vi "Read s4 channel status.vi"(8 "error in (no error)":errorcluster, 11 "SPARC4_Channel in":refnum<class "SPARC4_Channel.lvclass">) -> (0 "error out":errorcluster, 1 "channel status":T1, 2 "s4 channel status":T2, 3 "SPARC4_Channel out":refnum<class "SPARC4_Channel.lvclass">)   [LabVIEW 2018, in "SPARC4_Channel.lvclass"]
uses:
  SPARC4_Channel.lvclass
  SPARC4_Channel.lvclass/SPARC4_Channel.ctl
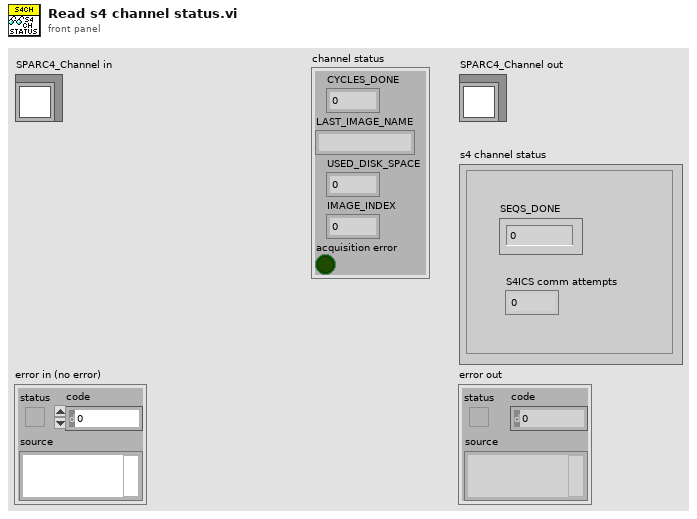
[diagram p1: front panel]
types:
  T1 = cluster{"CYCLES_DONE":u16, "LAST_IMAGE_NAME":string, "USED_DISK_SPACE":u16, "IMAGE_INDEX":u32, "acquisition error":bool}
  T2 = cluster{"SEQS_DONE":u16, "S4ICS comm attempts":u8}
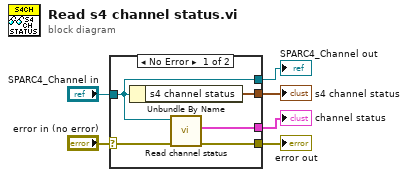
[diagram p0: block diagram]
diagram:
  n1 = case shown="No Error" "error in (no error)" {
    selector: "error in (no error)" -> [w9 w12]
    tunnel: [w8 w12] -> w5
    tunnel: [w10 w13] -> w3
    tunnel: "SPARC4_Channel in" -> [w10 w13]
    tunnel: [w11 _] -> w2
    tunnel: [w7 _] -> w1
    frame No Error {
      n2 = Unbundle By Name(w10) -> ("s4 channel status"=w11:T2)
      n3 = call-dynamic "Read channel status.vi"("error in (no error)"=w9, "Channel in"=w10) -> ("error out"=w8:errorcluster, "channel status"=w7:T1)  [unwired: 7 in, 1 out]
    }
    frame Error {
    }
  }
  "error out" <- w5
  "SPARC4_Channel out" <- w3
  "s4 channel status" <- w2
  "channel status" <- w1
